vi "CreateEvents.vi"(8 "error in (no error)":errorcluster) -> (0 "error out":errorcluster, 3 "Events":T1)   [LabVIEW 2022 SP3, in "Gui.lvlib" / "Gui.lvclass"]
uses:
  Gui.lvclass
  _Events.ctl
  Gui.lvclass/Gui.ctl
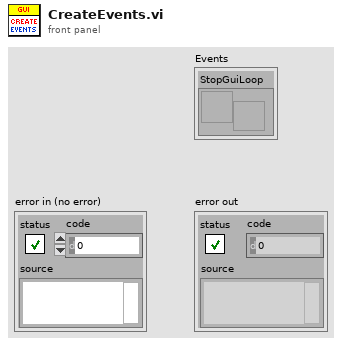
[diagram p1: front panel]
types:
  T1 = typedef "Gui.lvlib/Gui.lvclass/_Events.ctl" = cluster{"StopGuiLoop":refnum<user-event>}
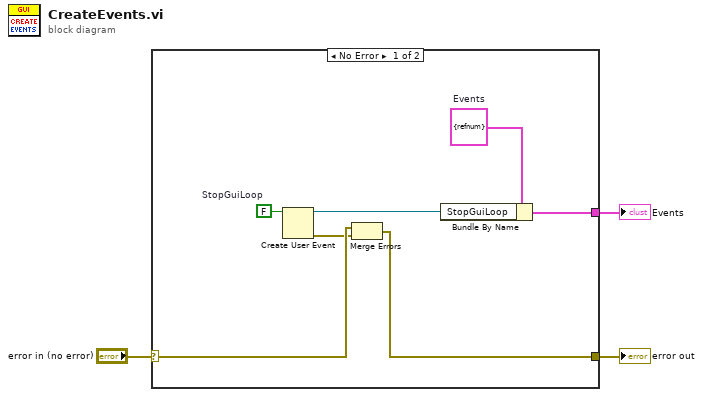
[diagram p0: block diagram]
diagram:
  n1 = case shown="No Error" "error in (no error)" {
    selector: "error in (no error)" -> [w5 w11]
    tunnel: [w7 w11] -> w2
    tunnel: [w6 _] -> w1
    frame No Error {
      w8 = T1 {"StopGuiLoop"=refnum}  # Events
      w10 = FALSE  # StopGuiLoop
      n2 = Create User Event(user event datatype=w10) -> (user event=w9:refnum<user-event>, error out=w4:errorcluster)  [unwired: 1 in]
      n3 = Merge Errors(w5, w4) -> (w7:errorcluster)
      n4 = Bundle By Name(cluster=w8, "StopGuiLoop"=w9) -> (w6:T1)
    }
    frame Error {
    }
  }
  "error out" <- w2
  "Events" <- w1
